vi "head_state_parse.vi"(4 "error in":errorcluster, 7 "msg in":string) -> (0 "error out":errorcluster, 1 "head_state":T2={"pan"=0.0, "isPanning"=FALSE, "isNodding"=TRUE}, 2 "Header":T1, 3 "msg out":string)   [LabVIEW 2015]
doc: "Parses a message into a head state"
uses:
  std_msgs/subs/parse_float64_scalar.vi
  std_msgs/subs/parse_bool_scalar.vi
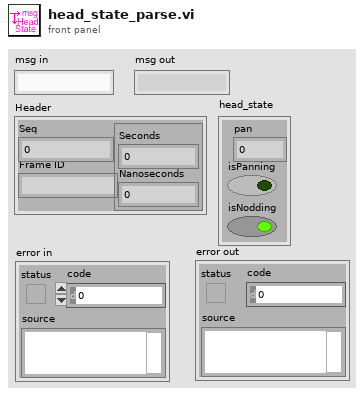
[diagram p1: front panel]
types:
  T1 = cluster{"Seq":u32, "Frame ID":string, "Timestamp":cluster{"Seconds":i32, "Nanoseconds":i32}}
  T2 = cluster{"pan":dbl, "isPanning":bool, "isNodding":bool}
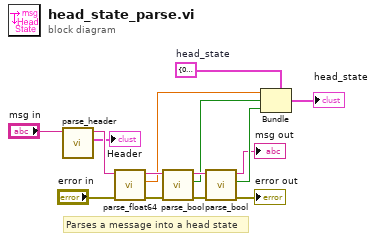
[diagram p0: block diagram]
diagram:
  w15 = T2 {"pan"=0.0, "isPanning"=TRUE, "isNodding"=TRUE}  # head_state
  # "Parses a message into a head state"
  n1 = call "parse_header.vi"("msg in"="msg in") -> ("Header"=→"Header":T1, "msg out"=w3:string)  [unwired: 4 in, 1 out]
  n2 = call-poly "parse_float64.vi"("error in"="error in", "msg in"=w3) -> ("error out"=w10:errorcluster, "number"=w5:dbl, "msg out"=w13:string)  [unwired: 3 in]
  n3 = call-poly "parse_bool.vi"("error in"=w10, "msg in"=w13) -> ("error out"=w9:errorcluster, "bool"=w6:bool, "msg out"=w12:string)  [unwired: 3 in]
  n4 = call-poly "parse_bool.vi"("error in"=w9, "msg in"=w12) -> ("error out"=→"error out":errorcluster, "bool"=w7:bool, "msg out"=→"msg out":string)  [unwired: 3 in]
  n5 = Bundle(cluster=w15, "pan"=w5, "isPanning"=w6, "isNodding"=w7) -> (→"head_state":T2)
